vi "Joystick Toggle.vi"(4 "Max":dbl, 6 "Min":dbl, 9 "Value":dbl, 11 "Range":dbl) -> (1 "Output":dbl)   [LabVIEW 2018]
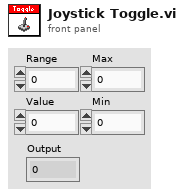
[diagram p1: front panel]
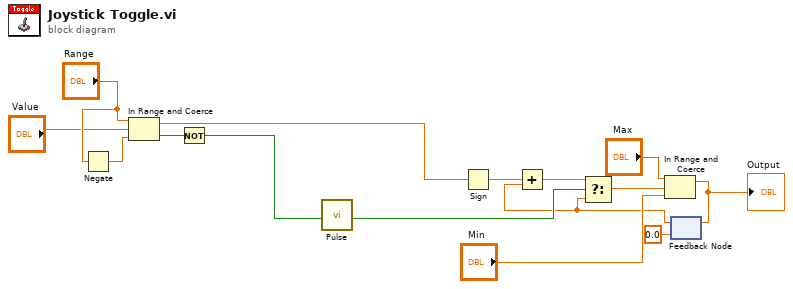
[diagram p0: block diagram]
diagram:
  n1 = Negate(x="Range") -> (-x=w13:dbl)
  n2 = In Range and Coerce(upper limit="Range", x="Value", lower limit=w13) -> (coerced(x)=w7:dbl, In Range?=w14:bool)
  n3 = Not(x=w14) -> (.not. x?=w15:bool)
  n4 = call "Pulse.vi"("Input"=w15) -> ("Output"=w9:bool)  [unwired: 10 in]
  n5 = Sign(1:w7) -> (0:w10:dbl)
  n6 = feedback #1(0.0 ("Max")) -> (w2:dbl)
  n7 = Add(x=w10, y=w2) -> (x+y=w8:dbl)
  n8 = Select(t=w8, s=w9, f=w2) -> (s? t:f=w6:dbl)
  n9 = In Range and Coerce(upper limit="Max", x=w6, lower limit="Min") -> (coerced(x)=w3:dbl)  [unwired: 1 out]
  "Output" <- w3
  n10 = feedback-in #1(w3) -> ()
